vi "Check Color Range Port.vi"(11 "Port Color Range":refnum<vi>) -> ()   [LabVIEW 2019]
uses:
  <vilib>/Rock Robotics/Network Tables/NT Read String.vi
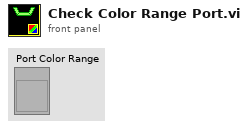
[diagram p1: front panel]
types:
  T1 = cluster{"Hue":cluster{dbl, dbl}, "Sat":cluster{dbl, dbl}, "Val":cluster{dbl, dbl}}
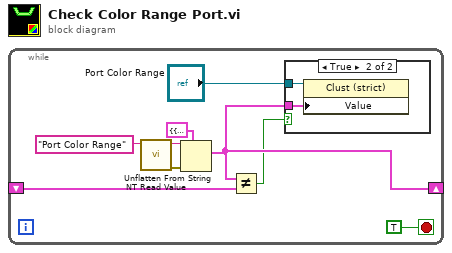
[diagram p0: block diagram]
diagram:
  n1 = while {
    shift-right: [w2] -> _
    shift-left: _ -> [w3]
    stop <- TRUE stop-if-true
    n2 = call-poly <vilib>:"NT Read Value.vi"("Name"="Port Color Range") -> ("error out"=w7:errorcluster, "String"=w8:string)  [unwired: 9 in]
    n3 = Unflatten From String(type=T1 {"Hue"={103.0, 151.0}, "Sat"={216.98804569244385, 255.0}, "Val"={201.0, 249.0}} ("Port Color Range"), binary string=w8, error in (no error)=w7) -> (value=w2:T1)  [unwired: 2 in, 2 out]
    n4 = Not Equal?(x=w2, y=w3) -> (x != y?=w1:bool)
    n5 = case shown="True" w1 {
      tunnel: "Port Color Range" -> [_ w11]
      tunnel: w2 -> [_ w10]
      frame False {
      }
      frame True {
        n6 = property on="Property Node" class="Clust (strict)"(reference=w11, "Value"=w10) -> ()  [unwired: 1 in, 2 out]
      }
    }
  }
